vi "Update Configuration.vi"(8 "error in (no error)":errorcluster, 10 "Parameters":T3, 11 "Comm Ref":T4) -> (0 "error out":errorcluster, 1 "Timed Out?":bool, 2 "GetSettings":T1, 3 "Comm Ref":T4)   [LabVIEW 2013, in "PID Control Host API.lvlib"]
uses:
  PID Control Host API.lvlib
  <vilib>/NI Veristand/Execution/CustomDevice/Custom Device Ref.ctl
  NationalInstruments.VeriStand.ClientAPI
  Shared/Types/Update Parameters Message.ctl
  Shared/Types/Get Settings Message.ctl
  Shared/Types/Gain Schedule.ctl
  <vilib>/NI Veristand/Execution/CustomDevice/NI VeriStand - Send Custom Device Message (String).vi
  Shared/Control Addon Shared.lvlib
  <vilib>/NI VeriStand/Execution/CustomDevice/NI_VS Custom Device ExecutionAPI.lvlib
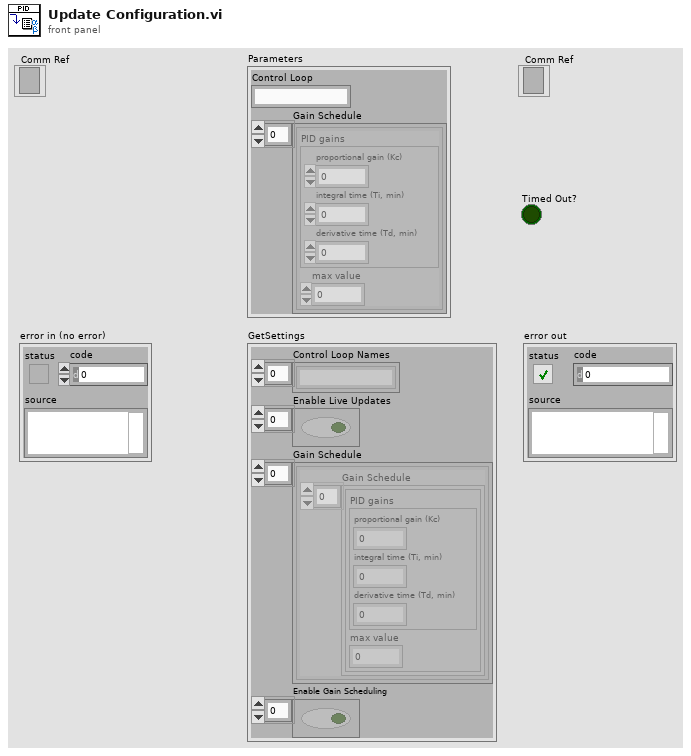
[diagram p1: front panel]
types:
  T1 = typedef "Control Addon Shared.lvlib/Get Settings Message.ctl" = cluster{"Control Loop Names":string[], "Enable Live Updates":bool[], "Gain Schedule":T2[], "Enable Gain Scheduling":bool[]}
  T2 = typedef "Control Addon Shared.lvlib/Gain Schedule.ctl" = cluster{"Gain Schedule":cluster{"PID gains":cluster{"proportional gain (Kc)":dbl, "integral time (Ti, min)":dbl, "derivative time (Td, min)":dbl}, "max value":dbl}[]}
  T3 = typedef "Control Addon Shared.lvlib/Update Parameters Message.ctl" = cluster{"Control Loop":string, "Gain Schedule":cluster{"PID gains":cluster{"proportional gain (Kc)":dbl, "integral time (Ti, min)":dbl, "derivative time (Td, min)":dbl}, "max value":dbl}[]}
  T4 = typedef "NI_VS Custom Device ExecutionAPI.lvlib/Custom Device Ref.ctl" = refnum<k24>
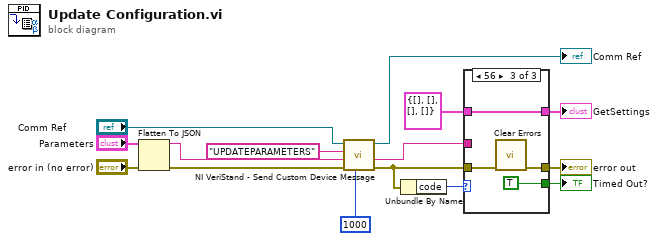
[diagram p0: block diagram]
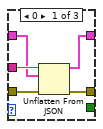
[diagram p2: hidden frame]
diagram:
  n1 = Flatten To JSON(anything="Parameters", error in (no error)="error in (no error)") -> (JSON string=w4:string, 11:w6:errorcluster)  [unwired: 1 in]
  n2 = call-poly <vilib>:"NI VeriStand - Send Custom Device Message.vi"("Timeout ms (5000)"=1000, "error in (no error)"=w6, "Data"=w4, "Command"="UPDATEPARAMETERS" ("Name"), "Custom Device in"="Comm Ref") -> ("error out"=w3:errorcluster, "Response"=w5:string, "Custom Device out"=→"Comm Ref":T4)  [unwired: 4 in]
  n3 = Unbundle By Name(w3) -> ("code"=w2:i32)
  n4 = case shown="56" w2 {
    tunnel: w5 -> [w20 _ _]
    tunnel: w3 -> [w19 w22 w23]
    tunnel: [w18 w22 w24] -> w12
    tunnel: [w17 w21 w26] -> w11
    tunnel: T1 {"Control Loop Names"=[], "Enable Live Updates"=[], "Gain Schedule"=[], "Enable Gain Scheduling"=[]} ("GetSettings") -> [w16 w21 w26]
    tunnel: [_ _ TRUE] -> w1
    frame 0 {
      n5 = Unflatten From JSON(JSON string=w20, type and defaults=w16, error in (no error)=w19) -> (value=w17:T1, error out=w18:errorcluster)  [unwired: 4 in]
    }
    frame Default {
    }
    frame 56 {
      n6 = call <vilib>:"Clear Errors.vi"("error in (no error)"=w23) -> ("error out"=w24:errorcluster)  [unwired: 6 in]
    }
  }
  "error out" <- w12
  "Timed Out?" <- w1
  "GetSettings" <- w11
